vi "TakeImagesAtCoords.vi"(0 "Image feed":T1(plugin-control), 1 "Path to save stave calib":path=path "E:/XYZstage+Camera_CollectedImages/12-22-2016/images", 5 "Set of Coordinates to Process":dbl[][](array[numeric]), 7 "XYZ .NET Refnum in":refnum<k24>, 9 "Axes Speeds [mm/s]":T2={"X Speed"=25.0, "Y Speed"=10.0, "Z Speed"=10.0}, 11 "error in":errorcluster, 12 "Time & Temperature Stamp":dbl[](array[numeric]), 13 "milliseconds to wait":u32=3500) -> (6 "Image Array":T1[](array[plugin-control])=["remote image 000000001396EDEC", "remote image 000000001392CD9C", "remote image 000000001392D204", "remote image 00000000139777D4", "remote image 000000001397783C", "image_5", "image_6", "image_7", "image_8", "image_9", "image_10", "image_11", "image_12", "image_13", "image_14", "image_15", "image_16", "image_17"], 8 "XYZ .NET Refnum out":refnum<k24>, 10 "Captured positions":dbl[][](array[numeric]), 15 "Error report":errorcluster)   [LabVIEW 2016]
uses:
  C:/Users/Aerotech/Documents/BNLStaveAssembly-blueprint/Bin/Aerotech.A3200.dll
  BNLStaveAssembly-blueprint/Bin/Aerotech.A3200.dll
  <vilib>/Utility/file.llb/Write Delimited Spreadsheet (DBL).vi
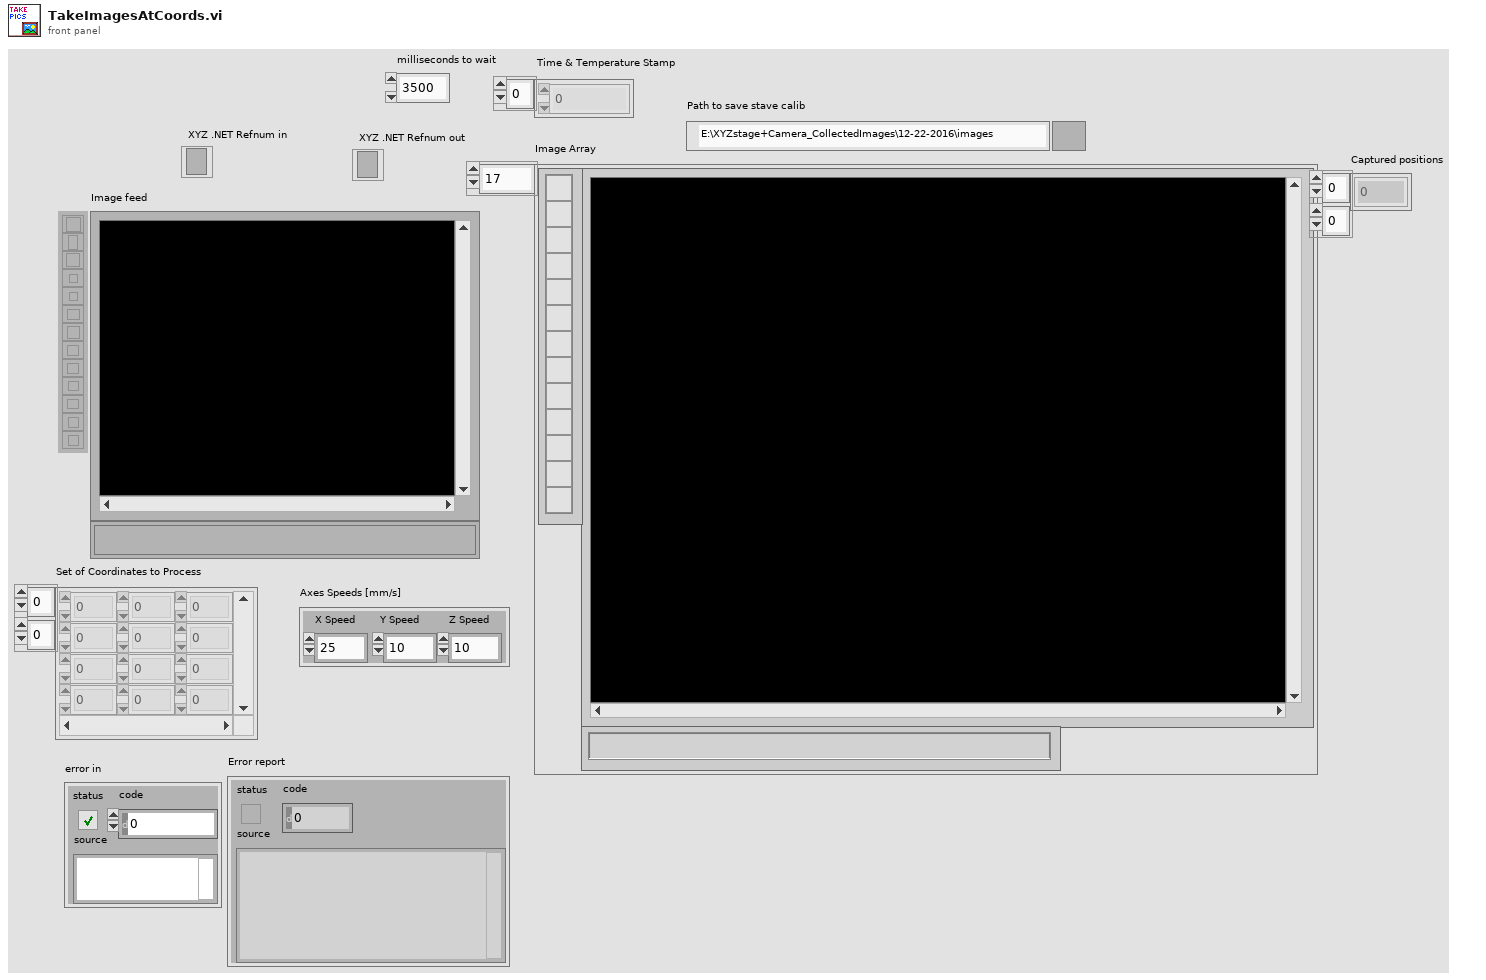
[diagram p1: front panel]
types:
  T1 = typedef "IMAQ Image.ctl" = refnum<image>
  T2 = cluster{"X Speed":dbl, "Y Speed":dbl, "Z Speed":dbl}
  T3 = cluster{"Image feed":T1, "Axes Speeds [mm/s]":cluster{"X Speed":dbl, "Y Speed":dbl, "Z Speed":dbl}, "XYZ .NET Refnum in":refnum<k24>}
  T4 = cluster{"Captured positions":dbl[][], "XYZ .NET Refnum out":refnum<k24>}
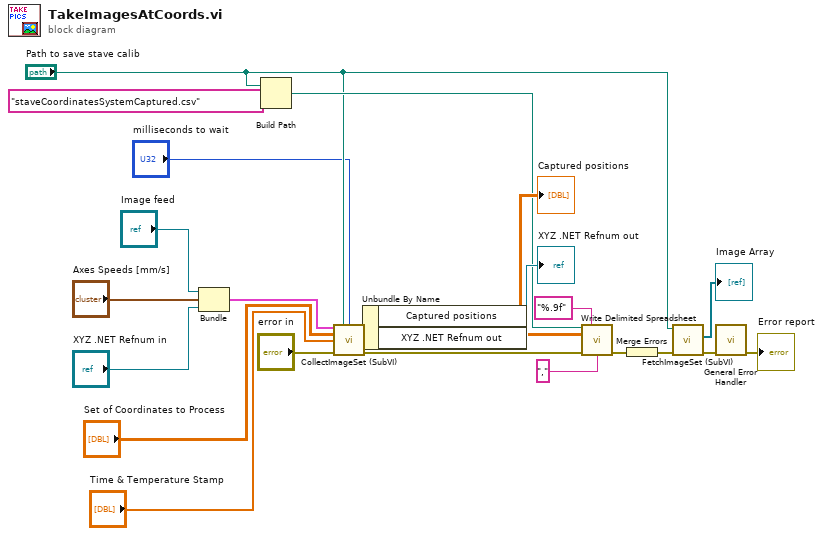
[diagram p0: block diagram]
diagram:
  n1 = Bundle("Image feed"="Image feed", "Axes Speeds [mm/s]"="Axes Speeds [mm/s]", "XYZ .NET Refnum in"="XYZ .NET Refnum in") -> (w2:T3)  [unwired: 1 in]
  n2 = Build Path(base path="Path to save stave calib", name or relative path="staveCoordinatesSystemCaptured.csv") -> (appended path=w5:path)
  n3 = call "CollectImageSet (SubVI).vi"("Inputs"=w2, "Path to save collected images"="Path to save stave calib", "milliseconds to wait"="milliseconds to wait", "Set of coordinates to process"="Set of Coordinates to Process", "Time & Temperature Stamp"="Time & Temperature Stamp", "error in"="error in") -> ("Outputs"=w12:T4, "error out"=w17:errorcluster)  [unwired: 7 in, 1 out]
  n4 = Unbundle By Name(w12) -> ("Captured positions"=w9:dbl[][], "XYZ .NET Refnum out"=→"XYZ .NET Refnum out":refnum<k24>)
  "Captured positions" <- w9
  n5 = call-poly <vilib>:"Write Delimited Spreadsheet.vi"("file path (dialog if empty)"=w5, "format (%.3f)"="%.9f", "2D data"=w9, "error in (no error)"=w17, "delimiter (\\t)"="," ("delimiter (\\t)")) -> ("error out"=w16:errorcluster)  [unwired: 9 in, 1 out]
  n6 = Merge Errors(w16) -> (w7:errorcluster)
  n7 = call "FetchImageSet (SubVI).vi"("error in (no error)"=w7, "Images Directory"="Path to save stave calib") -> ("error out"=w6:errorcluster, "Image Array"=→"Image Array":T1[])  [unwired: 7 in, 1 out]
  n8 = call <vilib>:"General Error Handler.vi"("error in (no error)"=w6) -> ("error out"=→"Error report":errorcluster)  [unwired: 2 in, 12 out]
